vi "HEX.vi"() -> ()   [LabVIEW 2020]
panel:
  out "Check Sum":i16 format="%x"
  in  "file path (use dialog)":path
  out "Text convert to Hex":string[](array[string])
  out "Text in Intel Hex":string
  out "Length of Text-Hex":string
  out "Length of Text-Decimal":i32
  in  "Text":string
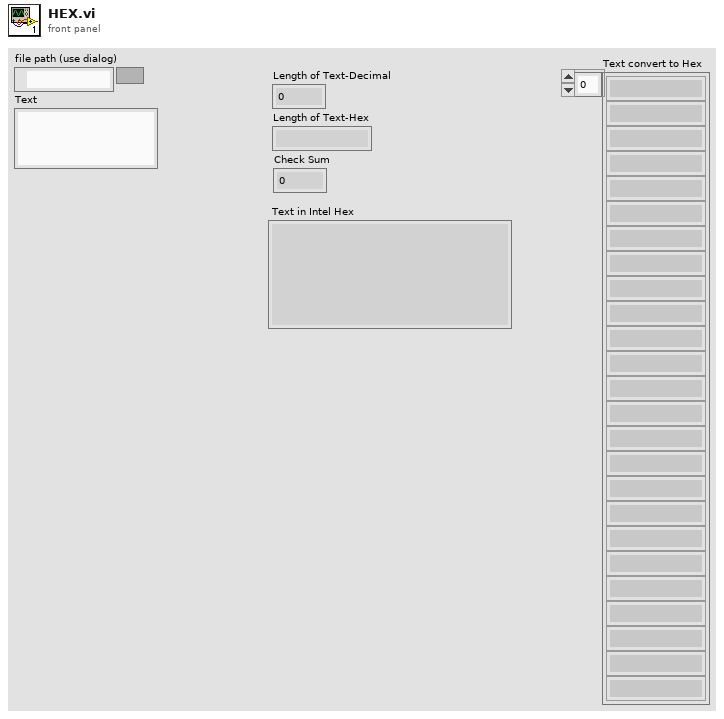
[diagram p1: front panel]
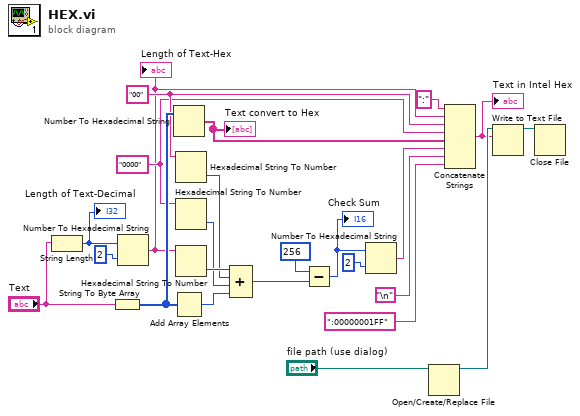
[diagram p0: block diagram]
diagram:
  w11 = "00" ("string")
  w10 = "0000"
  n1 = String Length(string="Text") -> (length=w24:i32)
  "Length of Text-Decimal" <- w24
  n2 = String To Byte Array(string="Text") -> (unsigned byte array=w22:u8[])
  n3 = Number To Hexadecimal String(1:i16 2 ("width (-)"), 2:w24) -> (0:w9:string)
  "Length of Text-Hex" <- w9
  n4 = Number To Hexadecimal String(2:w22) -> (0:w19:string[])  [unwired: 1 in]
  "Text convert to Hex" <- w19
  n5 = Add Array Elements(numeric array=w22) -> (sum=w5:u8)
  n6 = Hexadecimal String To Number(string=w11) -> (number=w7:u32)  [unwired: 2 in, 1 out]
  n7 = Hexadecimal String To Number(string=w10) -> (number=w6:u32)  [unwired: 2 in, 1 out]
  n8 = Hexadecimal String To Number(string=w9) -> (number=w8:u32)  [unwired: 2 in, 1 out]
  n9 = Compound Arithmetic op=ADD(w8, w7, w6, w5) -> (w1:u32)
  n10 = Subtract(x=i16 256, y=w1) -> (x-y=w3:i16)
  "Check Sum" <- w3
  n11 = Number To Hexadecimal String(1:i16 2 ("width (-)"), 2:w3) -> (0:w18:string)
  n12 = Open/Create/Replace File(file path (use dialog)="file path (use dialog)") -> (refnum out=w15:refnum<file>)  [unwired: 5 in, 2 out]
  n13 = Concatenate Strings(":", w9, w11, w10, w19, w18, "\n", ":00000001FF") -> (w13:string)
  "Text in Intel Hex" <- w13
  n14 = Write to Text File(file (use dialog)=w15, text=w13) -> (refnum out=w14:refnum<file>)  [unwired: 2 in, 2 out]
  n15 = Close File(refnum=w14) -> ()  [unwired: 1 in, 2 out]
